vi "IlluminatedG Better Search.vi"(6 "Variant in":variant, 7 "Shift Pressed?":bool, 8 "error in (no error)":errorcluster, 10 "QD Combo Box Ref":refnum<vi>, 11 "QD Launch VI Ref":refnum<vi>) -> (0 "error out":errorcluster, 4 "Variant out":variant)   [LabVIEW 2016]
doc: "Write a 1-2 sentence description of the functionality of your plugin here. Replace the \"$\" below with the character you wish to assign as the default shortcut for this plugin. Do not add any text after the 'Default Shortcut' line below.\n\nDefault Shortcut - [S]"
uses:
  IlluminatedG/Better Search/Data Types/Search Context.ctl
  IlluminatedG/Better Search/Better Search.lvlib
  IlluminatedG/Better Search/Data Types/Start Search Type.ctl
  IlluminatedG/Better Search/BetterSearch/BetterSearch.lvclass
  IlluminatedG/Better Search/Data Types/Type Reflection Item.ctl
  IlluminatedG/Better Search/Search/Search.lvclass
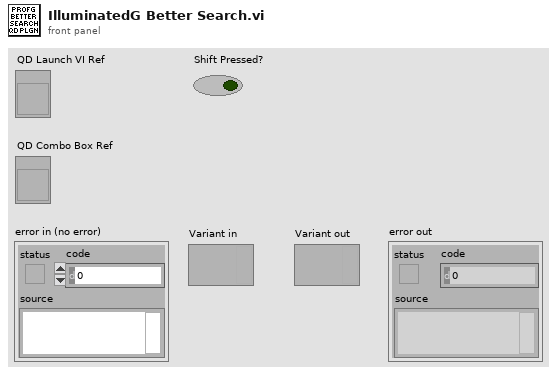
[diagram p1: front panel]
types:
  T1 = typedef "Better Search.lvlib/Start Search Type.ctl" = enum16{"Auto", "Text", "Data Type", "Bundle"}
  T2 = typedef "Better Search.lvlib/Search Context.ctl" = cluster{"Type ID":string, "VI Refnum":refnum<vi>, "Starting Text":string, "Shift?":bool, "App Ref":refnum<vi>, "Start Search Type":T1, "Item Graph":T3[], "Variant":variant}
  T3 = typedef "Better Search.lvlib/Type Reflection Item.ctl" = cluster{"Parent":i32, "Depth":i32, "Children":i32[], "Skip":bool, "Name":string, "Type":variant, "TypeID":string}
  T4 = typedef "Better Search.lvlib/Search Type Info.ctl" = cluster{"Search Type":T5, "Name":string, "Item":variant}
  T5 = typedef "Better Search.lvlib/Search Type.ctl" = enum16{"Generic", "Text", "Data Type", "VI", "Node"}
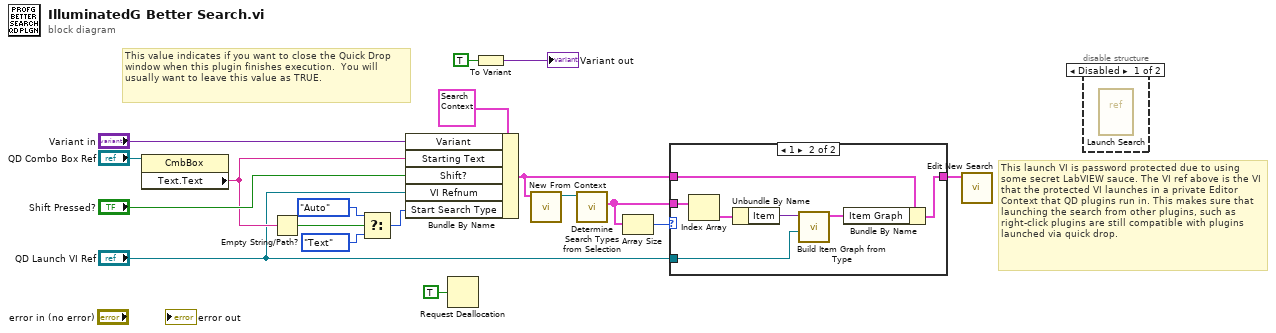
[diagram p0: block diagram]
diagram:
  # "This launch VI is password protected due to using some secret LabVIEW sauce. The VI ref above is the VI that the protected VI launches in a private Editor Context that QD plugins run in. This makes sure that launching the search from other plugins, such as right-click plugins are still compatible with plugins launched via quick drop."
  # "This value indicates if you want to close the Quick Drop window when this plugin finishes execution.  You will usually want to leave this value as TRUE."
  n1 = property class="CmbBox"(reference="QD Combo Box Ref") -> ("Text.Text"=w12:string)  [unwired: 1 in, 2 out]
  n2 = Empty String/Path?(string/path=w12) -> (empty?=w13:bool)
  n3 = Select(t=Start_Search_Type."Auto" ("Start Search Type"), s=w13, f=Start_Search_Type."Text" ("Start Search Type")) -> (s? t:f=w9:T1)
  n4 = Bundle By Name(cluster=T2 {"Type ID"="", "VI Refnum"=refnum, "Starting Text"="", "Shift?"=FALSE, "App Ref"=refnum, "Start Search Type"=enum."Auto", "Item Graph"=[], "Variant"=variant} ("Search Context"), "Variant"="Variant in", "Starting Text"=w12, "Shift?"="Shift Pressed?", "VI Refnum"="QD Launch VI Ref", "Start Search Type"=w9) -> (w4:T2)
  n5 = Request Deallocation(TRUE ("flag")) -> ()
  n6 = To Variant(anything=TRUE) -> (Variant=→"Variant out":variant)
  n7 = call "New From Context.vi"("Search Context"=w4) -> ("Search out"=w7:refnum<class "Search.lvclass">)  [unwired: 9 in, 1 out]
  n8 = call "Determine Search Types from Selection.vi"("Search in"=w7) -> ("Search Type Infos"=w5:T4[])  [unwired: 8 in, 2 out]
  n9 = Array Size(array=w5) -> (size(s)=w6:i32)
  n10 = case shown="1" w6 {
    tunnel: w5 -> [_ w26]
    tunnel: w4 -> [w19 w22]
    tunnel: "QD Launch VI Ref" -> [_ w23]
    tunnel: [w19 w20] -> w1
    frame Default {
    }
    frame 1 {
      n11 = Index Array(array=w26) -> (element=w25:T4)  [unwired: 1 in]
      n12 = Unbundle By Name(w25) -> ("Item"=w24:variant)
      n13 = call "Build Item Graph from Type.vi"("OwningVI"=w23, "Type"=w24) -> ("Item Graph"=w21:T3[])  [unwired: 8 in, 1 out]
      n14 = Bundle By Name(cluster=w22, "Item Graph"=w21) -> (w20:T2)
    }
  }
  n15 = call "Edit New Search.vi"("Search Context"=w1) -> ()  [unwired: 10 in, 1 out]
  n16 = disable-structure shown="Disabled" {
    frame Disabled {
      n17 = vi-ref "Launch Search.vi"() -> ()  [unwired: 1 out]
    }
    frame Enabled {
    }
  }
